vi "lqManifestation.vi"(8 "error in (no error)":errorcluster, 11 "LQObject in":refnum<class "LQObject.lvclass">) -> (0 "error out":errorcluster, 2 "Manifestation":u32, 3 "LQObject out":refnum<class "LQObject.lvclass">)   [LabVIEW 2013, in "Template.lvlib" / "LQObject.lvclass"]
uses:
  LQObject.lvclass
  LQObject.lvclass/LQObject.ctl
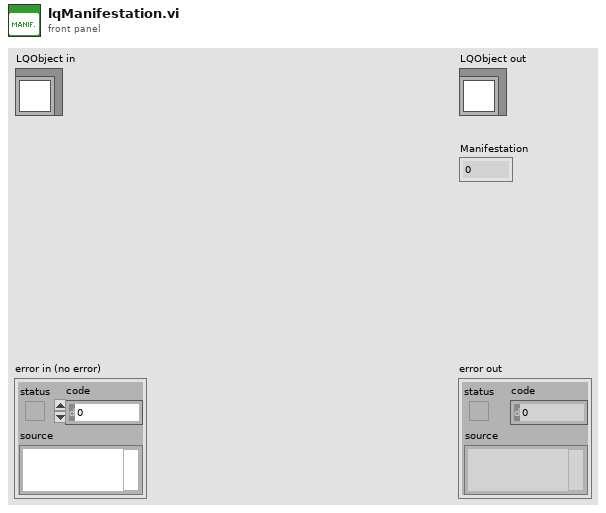
[diagram p1: front panel]
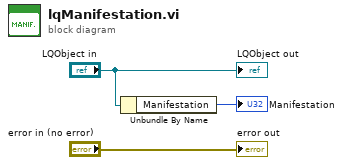
[diagram p0: block diagram]
diagram:
  n1 = Unbundle By Name("LQObject in") -> ("Manifestation"=→"Manifestation":u32)
  "error out" <- "error in (no error)"
  "LQObject out" <- "LQObject in"
